vi "check.cv_vols.last_modified.vi"(6 "Delay Time (2 sec)":dbl=2.0, 8 "error in (no error)":errorcluster, 11 "cv_vol paths":path[](array[path])) -> (0 "error out":errorcluster, 3 "Need Updating":path[](array[path]))   [LabVIEW 2024]
uses:
  WebScraper/comic_class/comic_class.lvclass
  WebScraper/comic_class/comic_class.lvclass/comic_class.ctl
  <vilib>/addons/_JKI.lib/Serialization/JSON/JKI JSON Serialization.lvlib
panel:
  out "current file":string
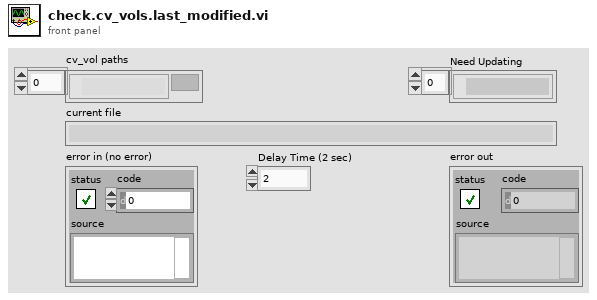
[diagram p1: front panel]
types:
  T1 = cluster{"date_last_updated":timestamp, "url":string}
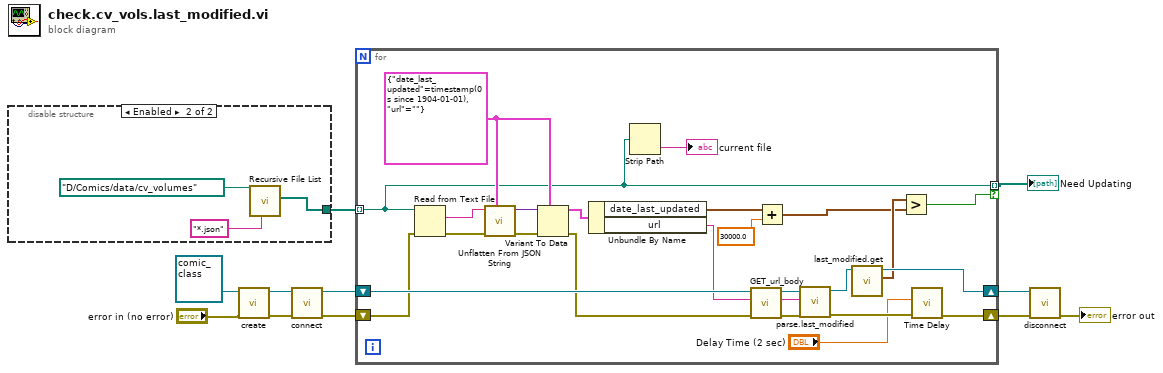
[diagram p0: block diagram]
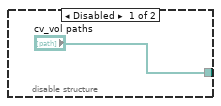
[diagram p2: hidden frame]
diagram:
  n1 = disable-structure shown="Enabled" {
    disable-tunnel: ["cv_vol paths" w15] -> w6
    frame Disabled {
    }
    frame Enabled {
      n2 = call <vilib>:"Recursive File List.vi"("pattern"="*.json", "Folder Path"=path "D:/Comics/data/cv_volumes") -> ("All Files in Dir"=w15:path[])  [unwired: 5 in, 4 out]
    }
  }
  n3 = call "create.vi"("error in (no error)"="error in (no error)", "comic_class in"=refnum<class "comic_class.lvclass"> refnum ("comic_class.lvclass")) -> ("error out"=w10:errorcluster, "comic_class out"=w9:refnum<class "comic_class.lvclass">)  [unwired: 8 in]
  n4 = call-dynamic "connect.vi"("error in (no error)"=w10, "comic_class in"=w9) -> ("error out"=w7:errorcluster, "comic_class out"=w8:refnum<class "comic_class.lvclass">)  [unwired: 8 in]
  n5 = for {
    shift-right: [w35] -> w3
    shift-left: w8 -> [w40]
    shift-right: [w26] -> w4
    shift-left: w7 -> [w34]
    tunnel: w6 -> [w23] mode=indexing
    tunnel: [w23] -> w5 mode=indexing if=w21
    w30 = T1 {"date_last_updated"=timestamp(0 s since 1904-01-01), "url"=""}
    n6 = Read from Text File(file (use dialog)=w23, error in=w34) -> (text=w31:string, error out=w29:errorcluster)  [unwired: 2 in, 2 out]
    n7 = call <vilib>:"Unflatten From JSON String.vi"("Type and Defaults"=w30, "error in"=w29, "JSON String"=w31) -> ("error out"=w33:errorcluster, "Variant"=w32:variant)  [unwired: 7 in]
    n8 = Variant To Data(error in=w33, type=w30, Variant=w32) -> (data=w27:T1, error out=w25:errorcluster)
    n9 = Unbundle By Name(w27) -> ("date_last_updated"=w18:timestamp, "url"=w24:string)
    n10 = Strip Path(path=w23) -> (name=→"current file":string)  [unwired: 1 out]
    n11 = call-dynamic "GET_url_body.vi"("error in (no error)"=w25, "url"=w24, "comic_class in"=w40) -> ("error out"=w37:errorcluster, "body"=w38:string, "comic_class out"=w39:refnum<class "comic_class.lvclass">)  [unwired: 6 in]
    n12 = Add(x=w18, y=30000.0) -> (x+y=w16:timestamp)
    n13 = call-dynamic "parse.last_modified.vi"("error in (no error)"=w37, "body"=w38, "comic_class in"=w39) -> ("error out"=w28:errorcluster, "comic_class out"=w36:refnum<class "comic_class.lvclass">)  [unwired: 7 in]
    n14 = call "last_modified.get.vi"("comic_class in"=w36) -> ("last modified"=w19:timestamp, "comic_class out"=w35:refnum<class "comic_class.lvclass">)  [unwired: 9 in]
    n15 = Greater?(x=w19, y=w16) -> (0:w21:bool)
    n16 = call "Time Delay"("error in (no error)"=w28, "Delay Time (s)"="Delay Time (2 sec)") -> ("error out"=w26:errorcluster)  [unwired: 9 in]
  }
  "Need Updating" <- w5
  n17 = call-dynamic "disconnect.vi"("error in (no error)"=w4, "comic_class in"=w3) -> ("error out"=→"error out":errorcluster)  [unwired: 8 in, 1 out]
